vi "replaceFieldTokens.vi"(8 "error in (no error)":errorcluster, 10 "Query In":string, 11 "BankingTransaction in":refnum<class "BankingTransaction.lvclass">) -> (0 "error out":errorcluster, 2 "Query Out":string, 3 "BankingTransaction out":refnum<class "BankingTransaction.lvclass">)   [LabVIEW 2018, in "BankingTransaction.lvclass"]
uses:
  BankingTransaction.lvclass
  BankingTransaction.lvclass/BankingTransaction.ctl
  Transaction/Transaction.lvclass
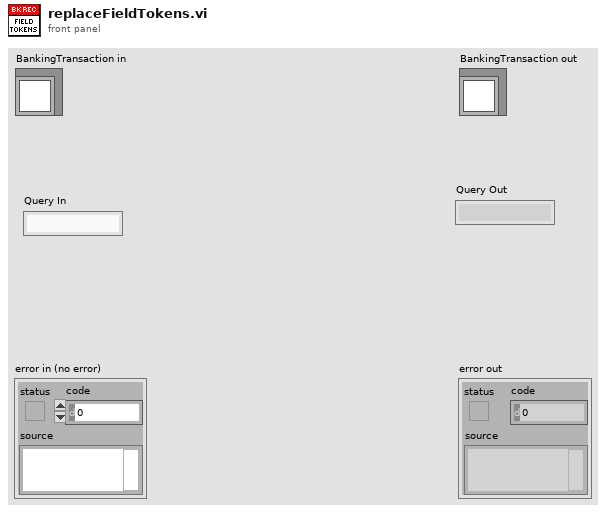
[diagram p1: front panel]
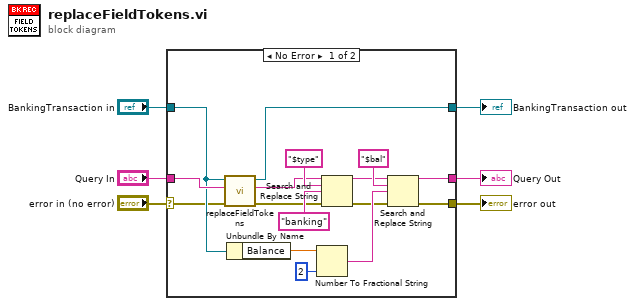
[diagram p0: block diagram]
diagram:
  n1 = case shown="No Error" "error in (no error)" {
    selector: "error in (no error)" -> [w7 w24]
    tunnel: [w22 w25] -> w6
    tunnel: "Query In" -> [w21 w23]
    tunnel: "BankingTransaction in" -> [w12 w25]
    tunnel: [w9 w24] -> w3
    tunnel: [w8 w23] -> w2
    frame No Error {
      n2 = call-parent "replaceFieldTokens.vi"("error in (no error)"=w7, "Query In"=w21, "Transaction in"=w12) -> ("error out"=w17:errorcluster, "Query Out"=w18:string, "Transaction out"=w22:refnum<class "BankingTransaction.lvclass">)  [unwired: 6 in]
      n3 = Unbundle By Name(w12) -> ("Balance"=w15:dbl)
      n4 = Number To Fractional String(number=w15, precision (6)=i16 2) -> (F-format string=w14:string)  [unwired: 2 in]
      n5 = Search and Replace String(input string=w18, search string="$type", replace string="banking" ("replace string (\"\")"), error in=w17) -> (result string=w11:string, error out=w10:errorcluster)  [unwired: 4 in, 2 out]
      n6 = Search and Replace String(input string=w11, search string="$bal", replace string=w14, error in=w10) -> (result string=w8:string, error out=w9:errorcluster)  [unwired: 4 in, 2 out]
    }
    frame Error {
    }
  }
  "error out" <- w3
  "BankingTransaction out" <- w6
  "Query Out" <- w2
